vi "Performance Test.vi"() -> ()   [LabVIEW 2021]
uses:
  ChannelCommon/typedef/Benchmark Stats.ctl
  CIFChannels/Typedef/Direction.ctl
  CIF_NIChn_Fifo_DAQ.lvclass
  D:/dev/Packages/Channel_Manager/src/CIFChannels/CIFChannels.lvclass
  D:/dev/Packages/Channel_Manager/src/CIF_NIChn/NIChn/CIF_NIChn.lvclass
  ChannelCommon/typedef/FIFO Config.ctl
  <vilib>/Platform/TimedLoop/XDataNode/timing_clust.ctl
  <vilib>/Platform/TimedLoop/XDataNode/nitl_modes.ctl
  <vilib>/Platform/TimedLoop/XDataNode/wakeup.ctl
  ChannelCommon/typedef/TimeStamps.ctl
  ChannelCommon/typedef/Datatype Waveform.ctl
  CIFChannels/CIFChannels.lvclass/CIFChannels.ctl
  CIF_NIChn_Fifo_DAQ.lvclass/CIF_NIChn_Fifo_DAQ.ctl
  NIChn/CIF_NIChn.lvclass/CIF_NIChn.ctl
  <vilib>/CIF Foundation/CIF Utilities/Statistics/I64/Stats_I64_CIF_U.lvclass/Stats_I64_CIF_U.ctl
  <vilib>/CIF Foundation/CIF Utilities/DataTypes/Flatten U64.vi
  SubVIs/Core Write DAQ FIFO.vi
  SubVIs/Core Read DAQ FIFO.vi
  <vilib>/CIF Foundation/CIF Utilities/Statistics/I64/Get Stats.vi
  ChannelCommon/Utilities/Reset Waveform DVRs.vi
  SubVIs/Core Write DAQ DVR FIFO.vi
  ChannelCommon/Utilities/Get Waveform DVRs.vi
  CIFChannels/Accessors/Read FIFO Retry on Timeout.vi
  SubVIs/Core Read DAQ FIFO.vi/a66d495f-c29f-4596-8ad9-13e7f334244d.vi
  SubVIs/Core Read DAQ FIFO.vi/010c5156-5ad7-4e56-b6b0-a69033aca011.vi
  CIFChannels/Utilities/Update Flatten Benchmark.vi
  SubVIs/Core Read DAQ DVR FIFO.vi
  <vilib>/CIF Foundation/CIF Channels/CIFChannels/Top Level/Write U8 Array.vi
  NIChn/Accessors/Read CIF Channel.vi
  NIChn/Accessors/Write CIF Channel.vi
  SubVIs/Flatten.vi
  CIFChannels/Accessors/Read FIFO Header.vi
  <vilib>/CIF Foundation/CIF Utilities/Time/System Time/Get System Time.vi
  <vilib>/CIF Foundation/CIF Utilities/Statistics/I64/X1 minus X0.vi
  NIChn/SubVIs/Check Disconnect.vi
  <vilib>/CIF Foundation/CIF Channels/CIFChannels/Top Level/Read U8 Array.vi
  ChannelCommon/Utilities/Unflatten Header.vi
  CIFChannels/Utilities/Update Channel Benchmark.vi
  SubVIs/Core Read DAQ DVR FIFO.vi/683dda70-af16-44bc-a524-9971cb6dbe1c.vi
  SubVIs/Core Read DAQ DVR FIFO.vi/9ab161bc-d75a-4f10-a981-8d657be3a6b1.vi
  CIFChannels/Accessors/Read Channel State.vi
  CIFChannels/Accessors/Read Direction.vi
  SubVIs/Unflatten.vi
  <vilib>/CIF Foundation/CIF Channels/CIFChannels/SubVIs/Get dll Path.vi
  <vilib>/CIF Foundation/CIF Channels/CIFChannels/SubVIs/Get Requested Size.vi
  ChannelCommon/CIFFIFO/Flatten/DVR Flatten.vi
  <vilib>/CIF Foundation/CIF Utilities/Time/System Time/LabVIEW Time to TAI Time.vi
  <vilib>/CIF Foundation/CIF Utilities/Statistics/I64/X1 minus X0.vi/dfabcf33-0dbc-4041-80a5-3dc0c86d2989.vi
  CIFChannels/Accessors/Write Channel State.vi
  CIFChannels/Accessors/Read Tag Disconnect Behavior.vi
  <vilib>/CIF Foundation/CIF Channels/CIFChannels/Top Level/Read U8 Array.vi/4bc1c15b-36ab-481f-b8dd-c64075ce723a.vi
  <vilib>/CIF Foundation/CIF Channels/CIFChannels/Top Level/Read U8 Array.vi/d83cb72b-7713-41fc-a3d1-682de79cf574.vi
  <vilib>/CIF Foundation/CIF Utilities/DataTypes/Unflatten U64.vi
  <vilib>/CIF Foundation/CIF Utilities/DataTypes/Unflatten I64.vi
  ChannelCommon/Utilities/Add Error.vi
  ChannelCommon/CIFFIFO/Flatten/DVR Unflatten.vi
  CIFChannels/Accessors/Write FIFO Header.vi
  CIFChannels/Accessors/Write FIFO Timeout.vi
  CIFChannels/Utilities/Create Flattened FIFO Header.vi
  <vilib>/CIF Foundation/CIF Utilities/Statistics/I64/X1 minus X0.vi/dfabcf33-0dbc-4041-80a5-3dc0c86d2989.vi/9eb60a9a-770f-4d2d-8b3f-8465c267ecc9.vi
  <vilib>/CIF Foundation/CIF Utilities/Errors/Append Error Location.vi
  ChannelCommon/Utilities/Flatten Header.vi
  CIFChannels/Utilities/Update FIFO Header.vi
  <vilib>/CIF Foundation/CIF Utilities/DataTypes/Flatten I64.vi
  NIChn/CIF_NIChn.lvclass
  <vilib>/Platform/TimedLoop/XDataNode/XDataNode.xnode
  <vilib>/Platform/TimedLoop/XDataNode/XDNodeRunTimeDep.lvlib
  CIFChannels/CIFChannels.lvclass
  ChannelCommon/ChannelCommon.lvlib
panel:
  out "Flatten (us) TO":T1
  out "Channel R/W (us) TO":T1
  out "Flatten (us)":T1
  out "Channel R/W (us)":T1
  out "avg TO":dbl
  out "max TO":dbl
  out "timed out? 3":bool
  out "timed out?":bool
  out "avg channel":dbl
  out "max channel":dbl
  out "pass":bool
  out "error out":errorcluster
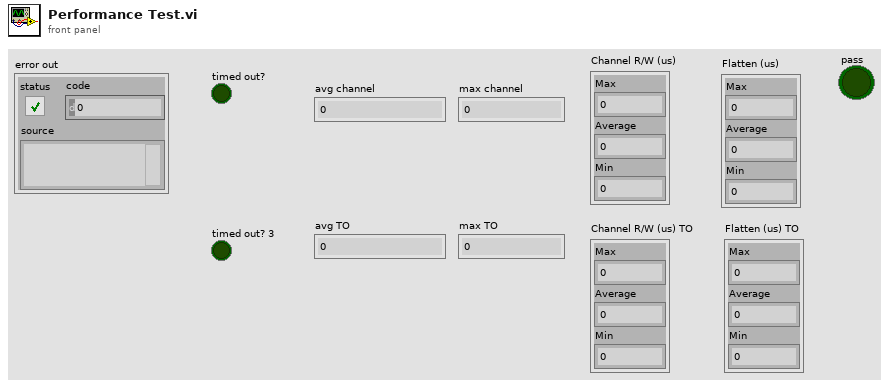
[diagram p1: front panel]
types:
  T1 = typedef "ChannelCommon.lvlib/Benchmark Stats.ctl" = cluster{"Max":i64, "Average":dbl, "Min":i64}
  T2 = typedef "ChannelCommon.lvlib/FIFO Config.ctl" = cluster{"Max Bytes/Msg":u64, "Max Msg/FIFO":u64, "Flags":u64}
  T3 = typedef "CIFChannels.lvclass/Direction.ctl" = enum16{"Publisher", "Subscriber"}
  T4 = typedef "ChannelCommon.lvlib/Datatype Waveform.ctl" = cluster{"measurement":dbl[], "dT":dbl, "Timestamp":i64, "Read Lock":bool}
  T5 = typedef "ChannelCommon.lvlib/TimeStamps.ctl" = cluster{"ClockID":u8, "T0":i64, "T_Out":i64}
  T6 = typedef "XDNodeRunTimeDep.lvlib/timing_clust.ctl" = cluster{"Expected End [f-1]":u64, "Actual End [f-1]":u64, "Finished Late? [f-1]":bool, "Expected End [i-1]":u64, "Actual End [i-1]":u64, "Finished Late? [i-1]":bool, "Expected Start [i]":u64, "Actual Start [i]":u64, "Expected Start [f]":u64, "Actual Start [f]":u64, "Source Name":string, "Structure Name":string, "Period":i64, "Deadline":i64, "Offset":i64, "Start":i64, "Priority":i32, "Timeout":i32, "Mode":T7, "Wakeup Reason":T8, "Error":errorcluster, "Source Type":string, "Secondary Source Type":string, "Global End Time":u64, "Global Start Time":u64, "Frame Duration":u64, "Iteration Duration":u64, "Assigned CPU":i32, "I/O Scan Engine Mode":u32}
  T7 = typedef "XDNodeRunTimeDep.lvlib/nitl_modes.ctl" = enum32{"No Change", "Process missed periods, maintain original phase", "Discard missed periods, maintain original phase", "Process missed periods, ignore original phase", "Discard missed periods, ignore original phase"}
  T8 = typedef "XDNodeRunTimeDep.lvlib/wakeup.ctl" = enum32{"Normal", "Aborted", "Asynchronous wakeup", "Timing source error", "Timed loop error", "Timeout"}
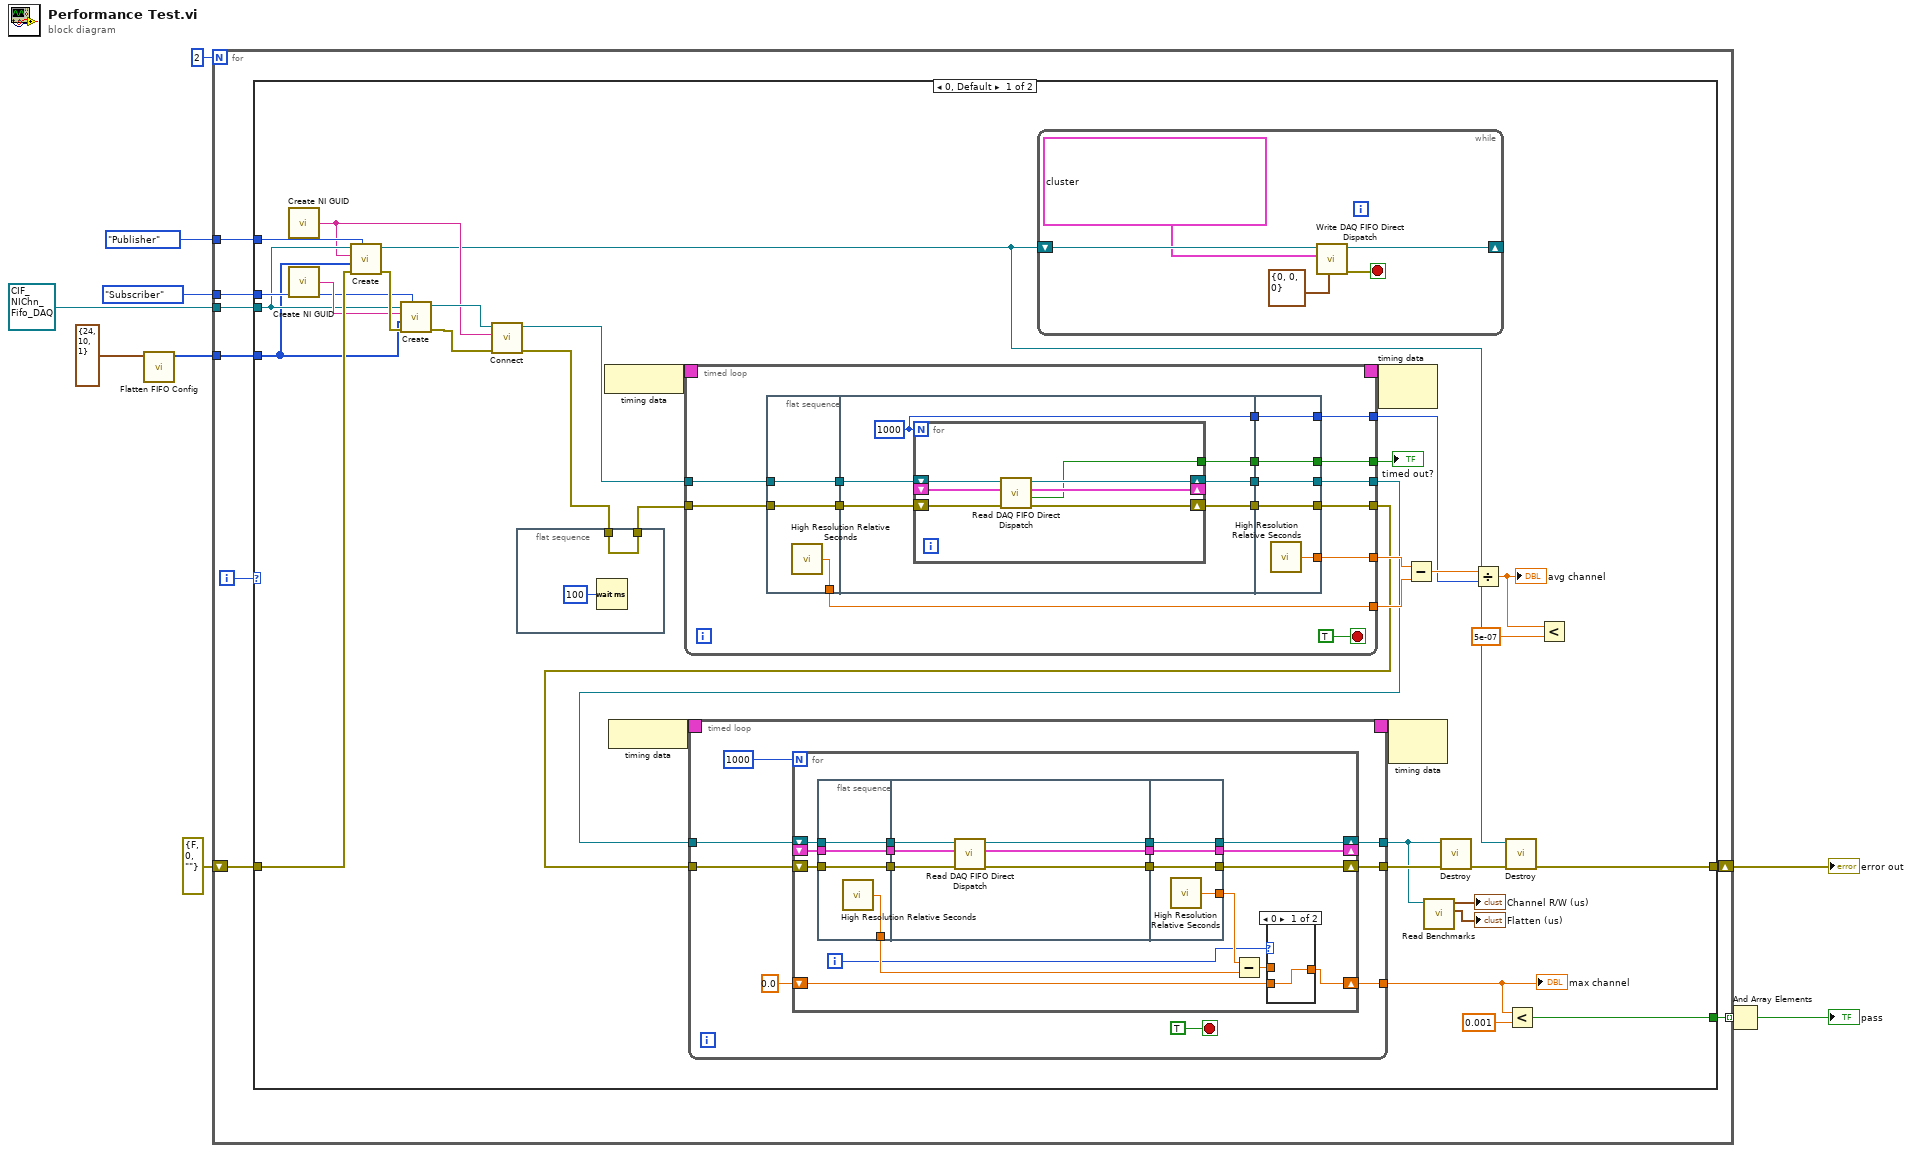
[diagram p0: block diagram]
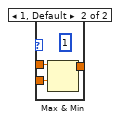
[diagram p2: hidden frame]
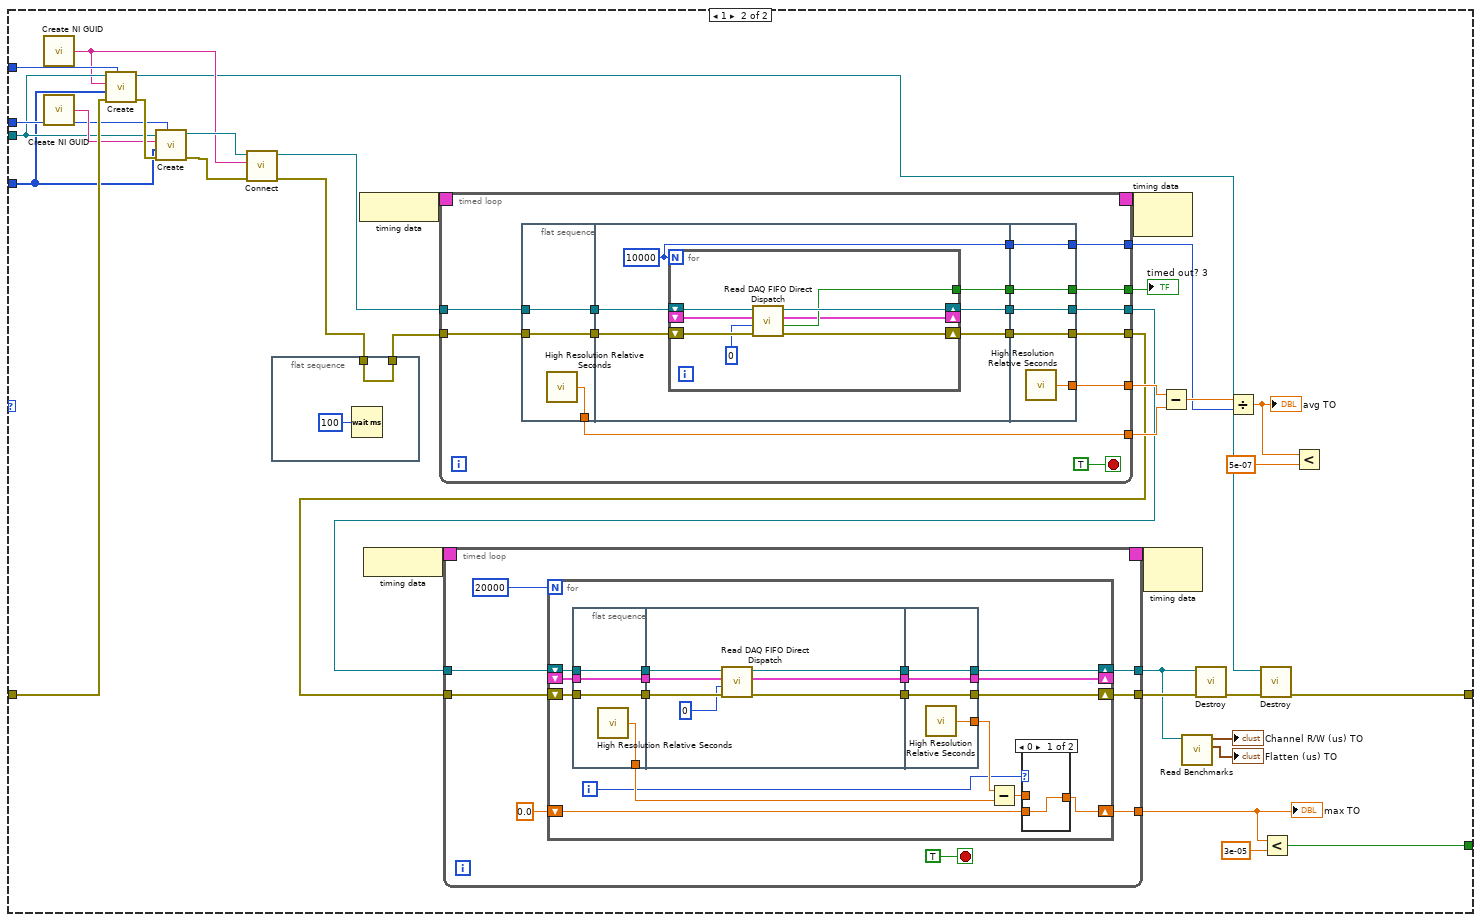
[diagram p3: hidden frame]
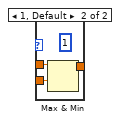
[diagram p4: hidden frame]
diagram:
  n1 = call "Flatten FIFO Config.vi"("FIFO Config in"=T2 {"Max Bytes/Msg"=24, "Max Msg/FIFO"=10, "Flags"=1}) -> ("Flattened FIFO Config"=w1:u8[])  [unwired: 10 in]
  n2 = for {
    N: 2 -> [_]
    tunnel: [w18] -> w8 mode=indexing
    shift-right: [w17] -> w10
    shift-left: errorcluster {"status"=FALSE, "code"=0, "source"=""} ("error out") -> [w15]
    tunnel: Direction."Publisher" ("Direction") -> [w14]
    tunnel: Direction."Subscriber" ("Direction") -> [w13]
    tunnel: refnum<class "CIF_NIChn_Fifo_DAQ.lvclass"> refnum ("CIF_NIChn_Fifo_Power.lvclass") -> [w12]
    tunnel: w1 -> [w11]
    i -> [w16]
    n3 = case shown="0, Default" w16 {
      tunnel: [w40 w171] -> w18
      tunnel: [w25 w156] -> w17
      tunnel: w15 -> [w38 w169]
      tunnel: w14 -> [w36 w167]
      tunnel: w13 -> [w35 w166]
      tunnel: w12 -> [w34 w165]
      tunnel: w11 -> [w30 w161]
      frame 0, Default {
        n4 = call <vilib>:"Create NI GUID.vi"() -> ("NI GUID"=w32:string)
        n5 = call <vilib>:"Create NI GUID.vi"() -> ("NI GUID"=w37:string)
        n6 = call-dynamic "Create.vi"("Direction"=w36, "error in (no error)"=w38, "Custom Config Data"=w30, "Name"=w32, "CIFTag in"=w34) -> ("error out"=w39:errorcluster, "CIFTag out"=w26:refnum<class "CIF_NIChn_Fifo_DAQ.lvclass">)  [unwired: 5 in]
        n7 = call-dynamic "Create.vi"("Direction"=w35, "error in (no error)"=w39, "Custom Config Data"=w30, "Name"=w37, "CIFTag in"=w34) -> ("error out"=w31:errorcluster, "CIFTag out"=w33:refnum<class "CIF_NIChn_Fifo_DAQ.lvclass">)  [unwired: 5 in]
        n8 = call-dynamic "Connect.vi"("error in (no error)"=w31, "Connection Name"=w32, "CIFTag in"=w33) -> ("error out"=w24:errorcluster, "CIFTag out"=w29:refnum<class "CIF_NIChn_Fifo_DAQ.lvclass">)  [unwired: 7 in]
        n9 = flat-sequence {
          tunnel: w24 -> [w56]
          tunnel: [w56] -> w23
          frame #0 {
            n10 = Wait (ms)(milliseconds to wait=u32 100) -> ()  [unwired: 1 out]
          }
        }
        n11 = node-c288() -> (w54:T6)
        n12 = node-c288() -> (w52:T6)
        n13 = timed-loop {
          timing: w54 -> [_]
          timing-out: [_] -> w53
          tunnel: w29 -> [w124]
          tunnel: w23 -> [w123]
          tunnel: [w119] -> w46
          tunnel: [w117] -> w45
          tunnel: [w115] -> w50
          tunnel: [w114] -> w49
          tunnel: [w113] -> w47
          tunnel: [w111] -> w22
          stop <- TRUE stop-if-true
          n14 = flat-sequence {
            tunnel: w123 -> [w126]
            tunnel: w124 -> [w127]
            tunnel: [w127] -> w121
            tunnel: [w126] -> w120
            tunnel: [w125] -> w114
            tunnel: w121 -> [w133]
            tunnel: w120 -> [w132]
            tunnel: [w131] -> w118
            tunnel: [w130] -> w116
            tunnel: [w129] -> w112
            tunnel: [w128] -> w110
            tunnel: [w145] -> w119
            tunnel: w118 -> [w145]
            tunnel: [w144] -> w117
            tunnel: w116 -> [w144]
            tunnel: [w143] -> w115
            tunnel: [w142] -> w113
            tunnel: w112 -> [w142]
            tunnel: [w141] -> w111
            tunnel: w110 -> [w141]
            frame #0 {
              n15 = call <vilib>:"High Resolution Relative Seconds.vi"() -> ("relative seconds"=w125:dbl)
            }
            frame #1 {
              w129 = 1000
              n16 = for {
                N: w129 -> [_]
                shift-right: [w135] -> w131
                shift-left: w133 -> [w140]
                shift-right: [w138] -> w130
                shift-left: w132 -> [w139]
                shift-right: [w137] -> _
                shift-left: _ -> [w136]
                tunnel: [w134] -> w128
                n17 = call "Read DAQ FIFO Direct Dispatch.vi"("error in (no error)"=w139, "DAQ In"=w136, "CIFTag in"=w140) -> ("error out"=w138:errorcluster, "timed out?"=w134:bool, "DAQ Out"=w137:T4[], "CIFTag out"=w135:refnum<class "CIF_NIChn_Fifo_DAQ.lvclass">)  [unwired: 4 in, 1 out]
              }
            }
            frame #2 {
              n18 = call <vilib>:"High Resolution Relative Seconds.vi"() -> ("relative seconds"=w143:dbl)
            }
          }
        }
        "timed out?" <- w22
        n19 = timed-loop {
          timing: w52 -> [_]
          timing-out: [_] -> w51
          tunnel: w46 -> [w69]
          tunnel: w45 -> [w68]
          tunnel: [w66] -> w21
          tunnel: [w65] -> w28
          tunnel: [w62] -> w42
          stop <- TRUE stop-if-true
          n20 = for {
            N: 1000 -> [_]
            shift-right: [w81] -> w66
            shift-left: w69 -> [w83]
            shift-right: [w80] -> w65
            shift-left: w68 -> [w82]
            shift-right: [w74] -> w62
            shift-left: 0.0 -> [w75]
            shift-right: [w73] -> _
            shift-left: _ -> [w79]
            i -> [w71]
            n21 = flat-sequence {
              tunnel: w82 -> [w94]
              tunnel: w83 -> [w95]
              tunnel: [w95] -> w87
              tunnel: [w94] -> w86
              tunnel: [w93] -> w77
              tunnel: w79 -> [w92]
              tunnel: [w92] -> w85
              tunnel: w87 -> [w101]
              tunnel: w86 -> [w100]
              tunnel: [w97] -> w84
              tunnel: w85 -> [w96]
              tunnel: [w98] -> w72
              tunnel: [w99] -> w70
              tunnel: [w105] -> w81
              tunnel: w84 -> [w105]
              tunnel: [w104] -> w80
              tunnel: [w103] -> w78
              tunnel: [w102] -> w73
              tunnel: w72 -> [w102]
              tunnel: w70 -> [w104]
              frame #0 {
                n22 = call <vilib>:"High Resolution Relative Seconds.vi"() -> ("relative seconds"=w93:dbl)
              }
              frame #1 {
                n23 = call "Read DAQ FIFO Direct Dispatch.vi"("error in (no error)"=w100, "DAQ In"=w96, "CIFTag in"=w101) -> ("error out"=w99:errorcluster, "DAQ Out"=w98:T4[], "CIFTag out"=w97:refnum<class "CIF_NIChn_Fifo_DAQ.lvclass">)  [unwired: 4 in, 2 out]
              }
              frame #2 {
                n24 = call <vilib>:"High Resolution Relative Seconds.vi"() -> ("relative seconds"=w103:dbl)
              }
            }
            n25 = Subtract(x=w78, y=w77) -> (x-y=w76:dbl)
            n26 = case shown="0" w71 {
              tunnel: w76 -> [_ w91]
              tunnel: w75 -> [w88 w90]
              tunnel: [w88 w89] -> w74
              frame 0 {
              }
              frame 1, Default {
                (unwired) u32 1 ("milliseconds to wait")
                n27 = Max & Min(x=w91, y=w90) -> (max(x,y)=w89:dbl)  [unwired: 1 out]
              }
            }
          }
        }
        "max channel" <- w42
        n28 = while {
          shift-right: [w58] -> _
          shift-left: w26 -> [w61]
          stop <- w59 stop-if-true
          n29 = call "Write DAQ FIFO Direct Dispatch.vi"("FIFO Timestamps"=T5 {"ClockID"=0, "T0"=0, "T_Out"=0}, "DAQ In"=T4[] [{"measurement"=array[200001 elements], "dT"=43.0, "Timestamp"=2, "Read Lock"=FALSE}, {"measurement"=array[200001 elements], "dT"=34.0, "Timestamp"=1, "Read Lock"=FALSE}], "CIFTag in"=w61) -> ("error out"=w59:errorcluster, "CIFTag out"=w58:refnum<class "CIF_NIChn_Fifo_DAQ.lvclass">)  [unwired: 5 in, 2 out]
        }
        n30 = node-c288(w53) -> ()  [unwired: 1 out]
        n31 = node-c288(w51) -> ()  [unwired: 1 out]
        n32 = Subtract(x=w50, y=w49) -> (x-y=w48:dbl)
        n33 = call "Read Benchmarks.vi"("CIFChannels in"=w21) -> ("Flatten (us)"=→"Flatten (us)":T1, "Channel R/W (us)"=→"Channel R/W (us)":T1)  [unwired: 9 in]
        n34 = call-dynamic "Destroy.vi"("error in (no error)"=w28, "CIF_NIChn_Fifo_Power_DVR in"=w21) -> ("error out"=w27:errorcluster)  [unwired: 8 in, 1 out]
        n35 = Divide(x=w48, y=w47) -> (x/y=w44:dbl)
        "avg channel" <- w44
        n36 = call-dynamic "Destroy.vi"("error in (no error)"=w27, "CIF_NIChn_Fifo_Power_DVR in"=w26) -> ("error out"=w25:errorcluster)  [unwired: 8 in, 1 out]
        n37 = Less?(x=w42, y=0.001) -> (x < y?=w40:bool)
        n38 = Less?(x=w44, y=5e-07) -> ()  [unwired: 1 out]
      }
      frame 1 {
        n39 = call <vilib>:"Create NI GUID.vi"() -> ("NI GUID"=w163:string)
        n40 = call <vilib>:"Create NI GUID.vi"() -> ("NI GUID"=w168:string)
        n41 = call-dynamic "Create.vi"("Direction"=w167, "error in (no error)"=w169, "Custom Config Data"=w161, "Name"=w163, "CIFTag in"=w165) -> ("error out"=w170:errorcluster, "CIFTag out"=w157:refnum<class "CIF_NIChn_Fifo_DAQ.lvclass">)  [unwired: 5 in]
        n42 = call-dynamic "Create.vi"("Direction"=w166, "error in (no error)"=w170, "Custom Config Data"=w161, "Name"=w168, "CIFTag in"=w165) -> ("error out"=w162:errorcluster, "CIFTag out"=w164:refnum<class "CIF_NIChn_Fifo_DAQ.lvclass">)  [unwired: 5 in]
        n43 = call-dynamic "Connect.vi"("error in (no error)"=w162, "Connection Name"=w163, "CIFTag in"=w164) -> ("error out"=w155:errorcluster, "CIFTag out"=w160:refnum<class "CIF_NIChn_Fifo_DAQ.lvclass">)  [unwired: 7 in]
        n44 = flat-sequence {
          tunnel: w155 -> [w187]
          tunnel: [w187] -> w154
          frame #0 {
            n45 = Wait (ms)(milliseconds to wait=u32 100) -> ()  [unwired: 1 out]
          }
        }
        n46 = node-c288() -> (w185:T6)
        n47 = node-c288() -> (w183:T6)
        n48 = timed-loop {
          timing: w185 -> [_]
          timing-out: [_] -> w184
          tunnel: w160 -> [w251]
          tunnel: w154 -> [w250]
          tunnel: [w246] -> w177
          tunnel: [w244] -> w176
          tunnel: [w242] -> w181
          tunnel: [w241] -> w180
          tunnel: [w240] -> w178
          tunnel: [w238] -> w153
          stop <- TRUE stop-if-true
          n49 = flat-sequence {
            tunnel: w250 -> [w253]
            tunnel: w251 -> [w254]
            tunnel: [w254] -> w248
            tunnel: [w253] -> w247
            tunnel: [w252] -> w241
            tunnel: w248 -> [w260]
            tunnel: w247 -> [w259]
            tunnel: [w258] -> w245
            tunnel: [w257] -> w243
            tunnel: [w256] -> w239
            tunnel: [w255] -> w237
            tunnel: [w273] -> w246
            tunnel: w245 -> [w273]
            tunnel: [w272] -> w244
            tunnel: w243 -> [w272]
            tunnel: [w271] -> w242
            tunnel: [w270] -> w240
            tunnel: w239 -> [w270]
            tunnel: [w269] -> w238
            tunnel: w237 -> [w269]
            frame #0 {
              n50 = call <vilib>:"High Resolution Relative Seconds.vi"() -> ("relative seconds"=w252:dbl)
            }
            frame #1 {
              w256 = 10000
              n51 = for {
                N: w256 -> [_]
                shift-right: [w265] -> w258
                shift-left: w260 -> [w268]
                shift-right: [w266] -> w257
                shift-left: w259 -> [w267]
                shift-right: [w263] -> _
                shift-left: _ -> [w262]
                tunnel: [w264] -> w255
                n52 = call "Read DAQ FIFO Direct Dispatch.vi"("error in (no error)"=w267, "Timeout (ms)"=0, "DAQ In"=w262, "CIFTag in"=w268) -> ("error out"=w266:errorcluster, "timed out?"=w264:bool, "DAQ Out"=w263:T4[], "CIFTag out"=w265:refnum<class "CIF_NIChn_Fifo_DAQ.lvclass">)  [unwired: 3 in, 1 out]
              }
            }
            frame #2 {
              n53 = call <vilib>:"High Resolution Relative Seconds.vi"() -> ("relative seconds"=w271:dbl)
            }
          }
        }
        "timed out? 3" <- w153
        n54 = timed-loop {
          timing: w183 -> [_]
          timing-out: [_] -> w182
          tunnel: w177 -> [w195]
          tunnel: w176 -> [w194]
          tunnel: [w192] -> w150
          tunnel: [w191] -> w159
          tunnel: [w188] -> w173
          stop <- TRUE stop-if-true
          n55 = for {
            N: 20000 -> [_]
            shift-right: [w207] -> w192
            shift-left: w195 -> [w209]
            shift-right: [w206] -> w191
            shift-left: w194 -> [w208]
            shift-right: [w200] -> w188
            shift-left: 0.0 -> [w201]
            shift-right: [w199] -> _
            shift-left: _ -> [w205]
            i -> [w197]
            n56 = flat-sequence {
              tunnel: w208 -> [w220]
              tunnel: w209 -> [w221]
              tunnel: [w221] -> w213
              tunnel: [w220] -> w212
              tunnel: [w219] -> w203
              tunnel: w205 -> [w218]
              tunnel: [w218] -> w211
              tunnel: w213 -> [w228]
              tunnel: w212 -> [w224]
              tunnel: [w227] -> w210
              tunnel: w211 -> [w225]
              tunnel: [w226] -> w198
              tunnel: [w223] -> w196
              tunnel: [w232] -> w207
              tunnel: w210 -> [w232]
              tunnel: [w231] -> w206
              tunnel: [w230] -> w204
              tunnel: [w229] -> w199
              tunnel: w198 -> [w229]
              tunnel: w196 -> [w231]
              frame #0 {
                n57 = call <vilib>:"High Resolution Relative Seconds.vi"() -> ("relative seconds"=w219:dbl)
              }
              frame #1 {
                n58 = call "Read DAQ FIFO Direct Dispatch.vi"("error in (no error)"=w224, "Timeout (ms)"=0, "DAQ In"=w225, "CIFTag in"=w228) -> ("error out"=w223:errorcluster, "DAQ Out"=w226:T4[], "CIFTag out"=w227:refnum<class "CIF_NIChn_Fifo_DAQ.lvclass">)  [unwired: 3 in, 2 out]
              }
              frame #2 {
                n59 = call <vilib>:"High Resolution Relative Seconds.vi"() -> ("relative seconds"=w230:dbl)
              }
            }
            n60 = Subtract(x=w204, y=w203) -> (x-y=w202:dbl)
            n61 = case shown="0" w197 {
              tunnel: w202 -> [_ w217]
              tunnel: w201 -> [w214 w216]
              tunnel: [w214 w215] -> w200
              frame 0 {
              }
              frame 1, Default {
                (unwired) u32 1 ("milliseconds to wait")
                n62 = Max & Min(x=w217, y=w216) -> (max(x,y)=w215:dbl)  [unwired: 1 out]
              }
            }
          }
        }
        "max TO" <- w173
        n63 = node-c288(w184) -> ()  [unwired: 1 out]
        n64 = node-c288(w182) -> ()  [unwired: 1 out]
        n65 = Subtract(x=w181, y=w180) -> (x-y=w179:dbl)
        n66 = call "Read Benchmarks.vi"("CIFChannels in"=w150) -> ("Flatten (us)"=→"Flatten (us) TO":T1, "Channel R/W (us)"=→"Channel R/W (us) TO":T1)  [unwired: 9 in]
        n67 = call-dynamic "Destroy.vi"("error in (no error)"=w159, "CIF_NIChn_Fifo_Power_DVR in"=w150) -> ("error out"=w158:errorcluster)  [unwired: 8 in, 1 out]
        n68 = Divide(x=w179, y=w178) -> (x/y=w175:dbl)
        "avg TO" <- w175
        n69 = call-dynamic "Destroy.vi"("error in (no error)"=w158, "CIF_NIChn_Fifo_Power_DVR in"=w157) -> ("error out"=w156:errorcluster)  [unwired: 8 in, 1 out]
        n70 = Less?(x=w173, y=3e-05) -> (x < y?=w171:bool)
        n71 = Less?(x=w175, y=5e-07) -> ()  [unwired: 1 out]
      }
    }
  }
  "error out" <- w10
  n72 = And Array Elements(Boolean array=w8) -> (logical AND=→"pass":bool)
